vi "Modify_VIPB_Display_Information.vi"   [LabVIEW 2021]
uses:
  <vilib>/JKI/VIPM API/command-line/support/VI Package Build Spec Data Cluster_vipm_api.ctl
  <vilib>/JKI/VIPM API/command-line/support/Version Info Cluster_vipm_api.ctl
  4199a0e4-84aa-42fd-b3f5-f9ce2ee7846d.vi
  <vilib>/JDP Science/JSONtext/JSON text to Variant.vi
  <vilib>/JDP Science/JSONtext/Variant to JSON Text.vi
  <vilib>/JDP Science/JSONtext/LVClass Serializer/JSONtext LVClass Serializer.lvclass
  <vilib>/Wiresmith Technology/G CLI/CLI Class/CLI.lvclass
  <vilib>/JKI/VIPM API/VIPM API_vipm_api.lvlib
types:
  T1 = enum32{"Invalid", "Standard", "Closed", "Hidden", "Minimized", "Maximized"}
  T2 = typedef "VIPM API_vipm_api.lvlib/VI Package Build Spec Data Cluster_vipm_api.ctl" = cluster{"Package Version":T3, "Product Name":string, "Company Name":string, "Author Name (Person or Company)":string, "Product Homepage (URL)":string, "Legal Copyright":string, "License Agreement Name":string, "Product Description Summary":string, "Product Description":string, "Release Notes - Change Log":string}
  T3 = typedef "VIPM API_vipm_api.lvlib/Version Info Cluster_vipm_api.ctl" = cluster{"major":u32, "minor":u32, "patch":u32, "build":u32}
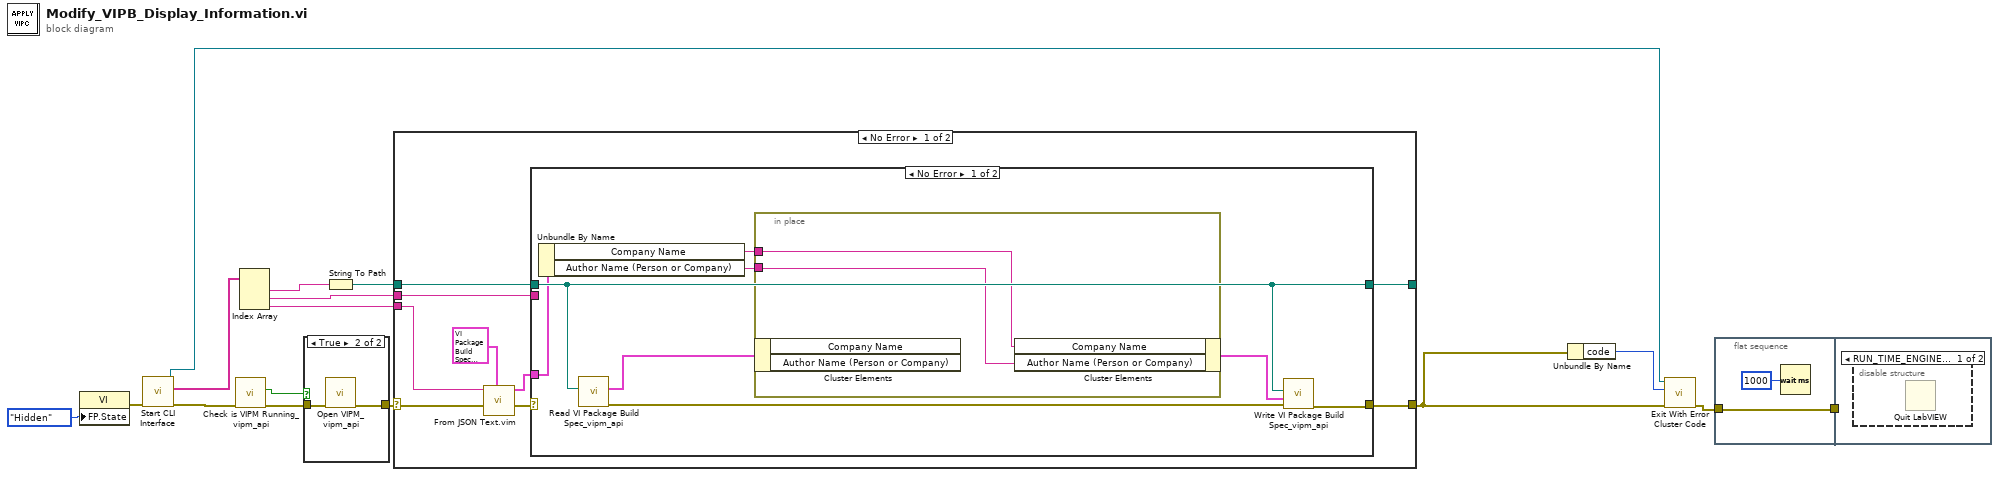
[diagram p0: block diagram]
diagram:
  n1 = property class="VI"("FP.State"=T1."Hidden" ("Front Panel Window:State")) -> (error out=w15:errorcluster)  [unwired: 2 in, 1 out]
  n2 = call <vilib>:"Start CLI Interface.vi"("error in (no error)"=w15) -> ("error out"=w7:errorcluster, "Custom Parameters"=w12:string[], "CLI out"=w14:refnum<class "CLI.lvclass">)  [unwired: 7 in, 1 out]
  n3 = call <vilib>:"Check is VIPM Running_vipm_api.vi"("error in (no error)"=w7) -> ("error out"=w13:errorcluster, "is Running"=w2:bool)  [unwired: 9 in]
  n4 = Index Array(array=w12) -> (element #1=w8:string, element #2=w3:string, element #3=w5:string)  [unwired: 3 in]
  n5 = case shown="True" w2 {
    tunnel: w13 -> [w17 w19]
    tunnel: [w17 w18] -> w6
    frame False {
    }
    frame True {
      n6 = call <vilib>:"Open VIPM_vipm_api.vi"("error in (no error)"=w19) -> ("error out"=w18:errorcluster)  [unwired: 10 in]
    }
  }
  n7 = String To Path(string=w8) -> (path=w4:path)
  n8 = case shown="No Error" w6 {
    selector: w6 -> [w28 w41]
    tunnel: w5 -> [w27 _]
    tunnel: w4 -> [w22 w40]
    tunnel: w3 -> [w21 _]
    tunnel: [w24 w41] -> w1
    tunnel: [w20 w40] -> _
    frame No Error {
      n9 = call "From JSON Text.vim"("Data Type and Default Value"=T2 {"Package Version"={"major"=0, "minor"=0, "patch"=0, "build"=0}, "Product Name"="", "Company Name"="", "Author Name (Person or Company)"="", "Product Homepage (URL)"="", "Legal Copyright"="", "License Agreement Name"="", "Product Description Summary"="", "Product Description"="", "Release Notes - Change Log"=""} ("VI Package Build Spec Data"), "error in (no error)"=w28, "JSON"=w27) -> ("error out"=w26:errorcluster, "Data out"=w23:T2)  [unwired: 7 in]
      n10 = case shown="No Error" w26 {
        tunnel: [w36 _] -> w24
        tunnel: w23 -> [w32 _]
        tunnel: w22 -> [w35 w39]
        tunnel: w21 -> [_ _]
        tunnel: [w35 w39] -> w20
        frame No Error {
          n11 = Unbundle By Name(w32) -> ("Company Name"=w31:string, "Author Name (Person or Company)"=w30:string)
          n12 = call <vilib>:"Read VI Package Build Spec_vipm_api.vi"("Path to VIPB File"=w35) -> ("error out"=w34:errorcluster, "VI Package Build Spec Data"=w33:T2)  [unwired: 9 in]
          n13 = in-place {
            in-place-border: w31 -> [w38]
            in-place-border: w30 -> [w37]
            n14 = in-place-cluster #1(w33) -> ()  [unwired: 2 out]
            n15 = in-place-cluster #1("Company Name"=w38, "Author Name (Person or Company)"=w37) -> (w29:T2)
          }
          n16 = call <vilib>:"Write VI Package Build Spec_vipm_api.vi"("error in (no error)"=w34, "VI Package Build Spec Data"=w29, "Path to VIPB File"=w35) -> ("error out"=w36:errorcluster)  [unwired: 8 in]
        }
        frame Error {
        }
      }
    }
    frame Error {
    }
  }
  n17 = Unbundle By Name(w1) -> ("code"=w9:i32)
  n18 = call <vilib>:"Exit With Error Cluster Code.vi"("error in (no error)"=w1, "No Error Code (0)"=w9, "CLI in"=w14) -> ("error out"=w10:errorcluster)  [unwired: 8 in]
  n19 = flat-sequence {
    tunnel: w10 -> [w43]
    tunnel: [w43] -> w11
    tunnel: w11 -> [_]
    frame #0 {
      n20 = Wait (ms)(milliseconds to wait=u32 1000) -> ()  [unwired: 1 out]
    }
    frame #1 {
      n21 = disable-structure shown="RUN_TIME_ENGINE==True" {
        frame condition #0 {
          n22 = Quit LabVIEW() -> ()  [unwired: 1 in]
        }
        frame condition #1 (active) {
        }
      }
    }
  }
